vi "Insert SubPanel.vi"(8 "error in (no error)":errorcluster, 10 "VI Ref":refnum<vi>, 11 "Subpanel Ref":refnum<vi>) -> (0 "error out":errorcluster)   [LabVIEW 2015]
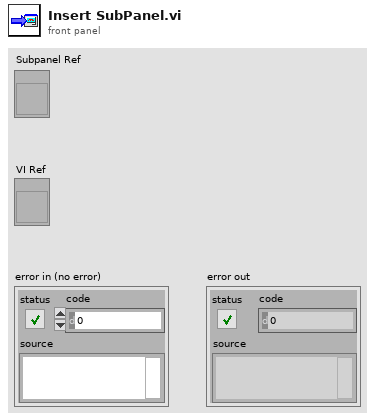
[diagram p1: front panel]
types:
  T1 = enum32{"Invalid", "Standard", "Closed", "Hidden", "Minimized", "Maximized"}
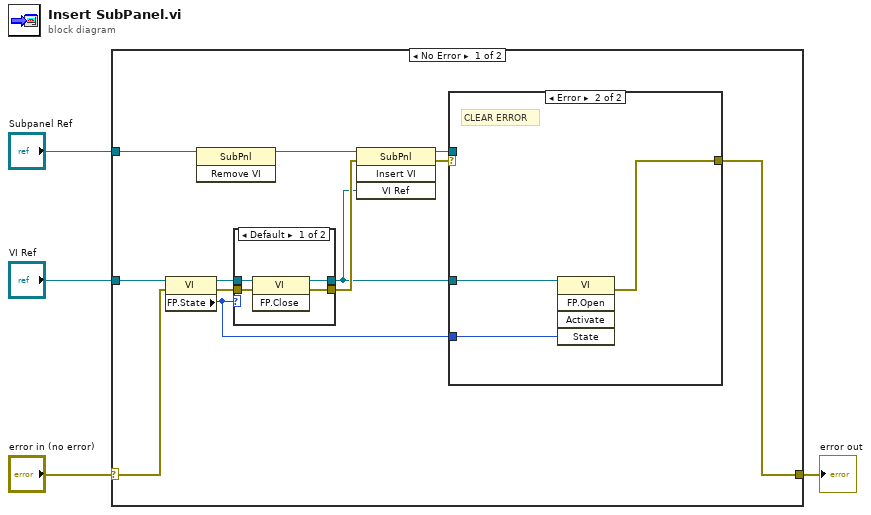
[diagram p0: block diagram]
diagram:
  n1 = case shown="No Error" "error in (no error)" {
    selector: "error in (no error)" -> [w8 w27]
    tunnel: "VI Ref" -> [w16 _]
    tunnel: "Subpanel Ref" -> [w6 _]
    tunnel: [w7 w27] -> w1
    frame No Error {
      n2 = property class="VI"(reference=w16, error in=w8) -> (reference out=w15:refnum<vi>, error out=w14:errorcluster, "FP.State"=w9:T1)
      n3 = invoke class="SubPnl" method="Remove VI"(reference=w6) -> (reference out=w5:refnum<vi>)  [unwired: 2 in, 2 out]
      n4 = case shown="Default" w9 {
        tunnel: w15 -> [w20 w22]
        tunnel: w14 -> [w19 w21]
        tunnel: [w18 w22] -> w10
        tunnel: [w17 w21] -> w13
        frame Default {
          n5 = invoke class="VI" method="FP.Close"(reference=w20, error in=w19) -> (reference out=w18:refnum<vi>, error out=w17:errorcluster)  [unwired: 1 in, 1 out]
        }
        frame "Closed" {
        }
      }
      n6 = invoke class="SubPnl" method="Insert VI"(reference=w5, error in=w13, "VI Ref"=w10) -> (reference out=w11:refnum<vi>, error out=w12:errorcluster)  [unwired: 1 in, 2 out]
      n7 = case shown="Error" w12 {
        selector: w12 -> [w23 _]
        tunnel: w11 -> [_ _]
        tunnel: w10 -> [_ w26]
        tunnel: w9 -> [_ w25]
        tunnel: [w23 w24] -> w7
        frame No Error {
        }
        frame Error {
          # "CLEAR ERROR"
          n8 = invoke class="VI" method="FP.Open"(reference=w26, "State"=w25) -> (error out=w24:errorcluster)  [unwired: 3 in, 4 out]
        }
      }
    }
    frame Error {
    }
  }
  "error out" <- w1
